vi "Element Init.vi"(7 "VolatusAPI":refnum<class "VolatusAPI.lvclass">, 8 "error in (no error)":errorcluster, 10 "JSON":string, 11 "NumericMatchBooleanIndicator in":refnum<class "NumericRangeBooleanIndicator.lvclass">) -> (0 "error out":errorcluster, 3 "NumericMatchBooleanIndicator out":refnum<class "NumericRangeBooleanIndicator.lvclass">)   [LabVIEW 2020, in "VolatusGUIElements.lvlib" / "NumericRangeBooleanIndicator.lvclass"]
uses:
  NumericRangeBooleanIndicator.lvclass
  Volatus/VolatusAPI/VolatusAPI.lvclass
  lv-vecto/Vecto/Group DBL/Group DBL.lvclass
  C:/dev/lv20CE/relink/lv-vecto/Vecto/Group/Group.lvclass
  JSON.ctl
  NumericRangeBooleanIndicator.lvclass/NumericRangeBooleanIndicator.ctl
  098e9b80-6dc1-4a73-92c4-25ef3c419290.vi
  <vilib>/JDP Science/JSONtext/JSON text to Variant.vi
  <vilib>/JDP Science/JSONtext/LVClass Serializer/JSONtext LVClass Serializer.lvclass
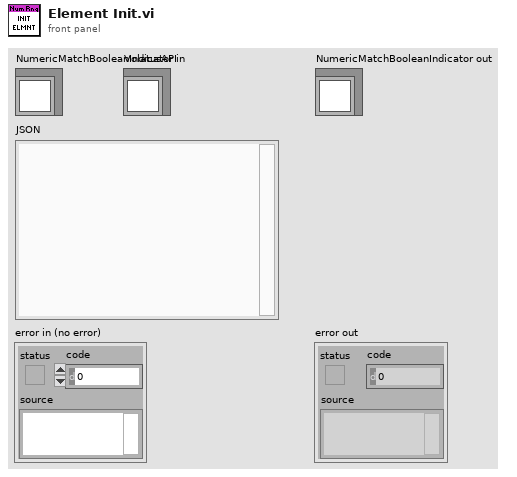
[diagram p1: front panel]
types:
  T1 = typedef "VolatusGUIElements.lvlib/NumericRangeBooleanIndicator.lvclass/JSON.ctl" = cluster{"Channel":string, "Low":dbl, "High":dbl}
  T2 = typedef "VectoConfig.lvlib/Channel Info.ctl" = cluster{"Name":string, "Group":string, "Owning Node":string, "Owning Task":string, "Resource":string}
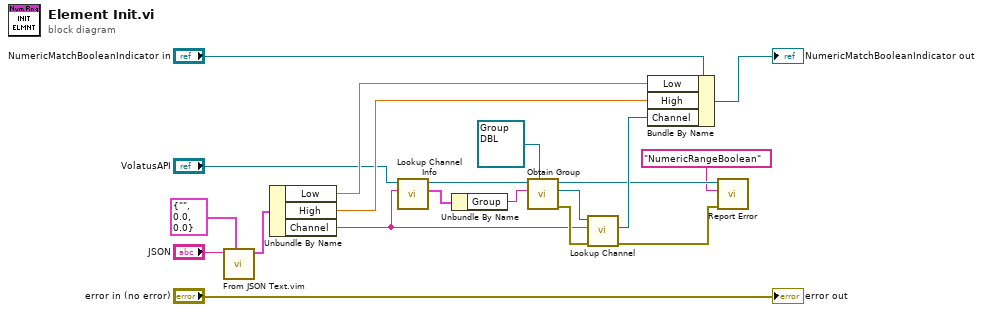
[diagram p0: block diagram]
diagram:
  n1 = call "From JSON Text.vim"("Data Type and Default Value"=T1 {"Channel"="", "Low"=0.0, "High"=0.0} ("JSON"), "JSON"="JSON") -> ("Data out"=w13:T1)  [unwired: 8 in, 1 out]
  n2 = Unbundle By Name(w13) -> ("Low"=w7:dbl, "High"=w8:dbl, "Channel"=w12:string)
  n3 = call "Lookup Channel Info.vi"("Channel Name"=w12, "VolatusAPI in"="VolatusAPI") -> ("Channel Info"=w15:T2, "VolatusAPI out"=w16:refnum<class "VolatusAPI.lvclass">)  [unwired: 6 in, 2 out]
  n4 = Unbundle By Name(w15) -> ("Group"=w14:string)
  n5 = call "Obtain Group.vi"("Group Type (Abstract)"=refnum<class "Group DBL.lvclass"> refnum ("Group in"), "Group Name"=w14, "VolatusAPI in"=w16) -> ("error out"=w19:errorcluster, "Group"=w17:refnum<class "Group DBL.lvclass">, "VolatusAPI out"=w3:refnum<class "VolatusAPI.lvclass">)  [unwired: 6 in]
  n6 = call "Lookup Channel.vi"("error in (no error)"=w19, "Channel Name"=w12, "Group in"=w17) -> ("error out"=w2:errorcluster, "Channel"=w11:refnum<class "Channel DBL.lvclass">)  [unwired: 6 in, 1 out]
  n7 = Bundle By Name(cluster="NumericMatchBooleanIndicator in", "Low"=w7, "High"=w8, "Channel"=w11) -> (→"NumericMatchBooleanIndicator out":refnum<class "NumericRangeBooleanIndicator.lvclass">)
  n8 = call "Report Error.vi"("error in (no error)"=w2, "Context"="NumericRangeBoolean", "VolatusAPI in"=w3) -> ()  [unwired: 7 in, 2 out]
  "error out" <- "error in (no error)"
